vi "prueba.vi"() -> ()   [LabVIEW 2016]
uses:
  <vilib>/userdefined/High Color/IMAQdx.ctl
  <vilib>/UPVI/lvhdf5/file.llb/LVH5F Operation.ctl
  C:/Users/Posgrado/Desktop/Rotational Stage/Thorlabs.MotionControl.Controls.dll
  Rotational Stage/Thorlabs.MotionControl.Controls.dll
  C:/Users/Posgrado/Desktop/Rotational Stage/Thorlabs.MotionControl.IntegratedStepperMotorsCLI.dll
  Rotational Stage/Thorlabs.MotionControl.IntegratedStepperMotorsCLI.dll
  <vilib>/Utility/miscctls.llb/LVRectTypeDef.ctl
  <vilib>/UPVI/lvhdf5/group.llb/H5G_obj_t.ctl
  <vilib>/UPVI/lvhdf5/dataset.llb/LVH5D Operation.ctl
  <vilib>/Analysis/baseanly.llb/Mean (DBL).vi
  <vilib>/UPVI/lvhdf5/group.llb/OpenCreateGroup (String).vi
  <vilib>/UPVI/lvhdf5/utility.llb/Select HDF5 Dialog.vi
  <vilib>/UPVI/lvhdf5/utility.llb/Select HDF5 Dialog (Object Only).vi
  <vilib>/UPVI/lvhdf5/dataset.llb/Simple H5Dwrite (Variant).vi
  <vilib>/UPVI/lvhdf5/library.llb/HDF5 Ref.ctl
  <vilib>/UPVI/lvhdf5/dataset.llb/Simple H5Dwrite.xnode
  <vilib>/vision/driver/NI_Vision_Acquisition_Software.lvlib
  <instrlib>/Keithley 2200 Series/Keithley 2200 Series.lvlib
  <vilib>/Analysis/NI_AALBase.lvlib
  <vilib>/UPVI/lvhdf5/identifier.llb/Not an HDF5 Refnum Constant.vi
  <vilib>/Utility/error.llb/Error Cluster From Error Code.vi
  <vilib>/UPVI/lvhdf5/dataset.llb/OpenCreateReplace Dataset by Element Type.vi
  <vilib>/UPVI/lvhdf5/dataspace.llb/H5Sselect_hyperslab.vi
  <vilib>/UPVI/lvhdf5/dataset.llb/H5Dwrite (Variant).vi
  <vilib>/UPVI/lvhdf5/dataset.llb/H5Dget_space.vi
  <vilib>/UPVI/lvhdf5/attribute.llb/private/LVH5AwriteWDTAttrs.vi
  <vilib>/UPVI/lvhdf5/dataspace.llb/H5Sclose.vi
  <vilib>/UPVI/lvhdf5/dataset.llb/H5Dclose.vi
  <vilib>/UPVI/lvhdf5/utility.llb/Select HDF5 Dialog (File and Object).vi
panel:
  in  "path":path
  out "Ángulo del polarizador":i32
  in  "CageRotatorControl":refnum<k24>(container)
  in  "SerialNumber":string="55000538"
  in  "Ring":u16(ring)
  out "I-V":cluster{dbl[], dbl[]}(graph)
  out "corriente":dbl
  in  "stop medición":bool
  in  "stop":bool
  in  "Iniciar medición":bool
  out "Readout value":dbl format="%^#_9e"
  out "LockIn":dbl
  out "Valor voltaje":dbl
  in  "Config. fotodiodo":cluster{"tiempo. lect.":dbl, "num. med":dbl}
  in  "Powermeter":T1={"Readout Config"="POW", "tiempo. lect."=0.0, "average rate"=0.0}
  in  "config. Polarizador":T2
  in  "Config. voltaje y corriente":T3 {"Measurement Function (0:Voltage)" items=["Voltage", "Current", "Power"]; "Unit(V)" items=["V", "mV", "kV", "A", "mA"]; "Function(0:Voltage)" items=["Voltage", "Current"]}
  in  "yFin":dbl
  in  "Paso":dbl=0.01
  in  "xFin":dbl
  in  "Movimiento de spot en x":ext(slide) scale=-10.0..10.0
  in  "Movimiento de spot en y":dbl(slide) min=-10.0 max=10.0 scale=-10.0..10.0
  out "xsal":dbl
  out "ysal":dbl
  in  "tipo":enum16{"barrido", "manual"}(ring)
  out "Fototubo":cluster{dbl[], dbl[]}(graph)
  out "Power meter":cluster{dbl[], dbl[]}(graph)
  out "Imágen":T4(plugin-control)
  out "flags":bool[](array[boolean])
  out "name":string
  out "Readout string":string
  out "New":bool
  out "Error log":string
  # "Control espejos"
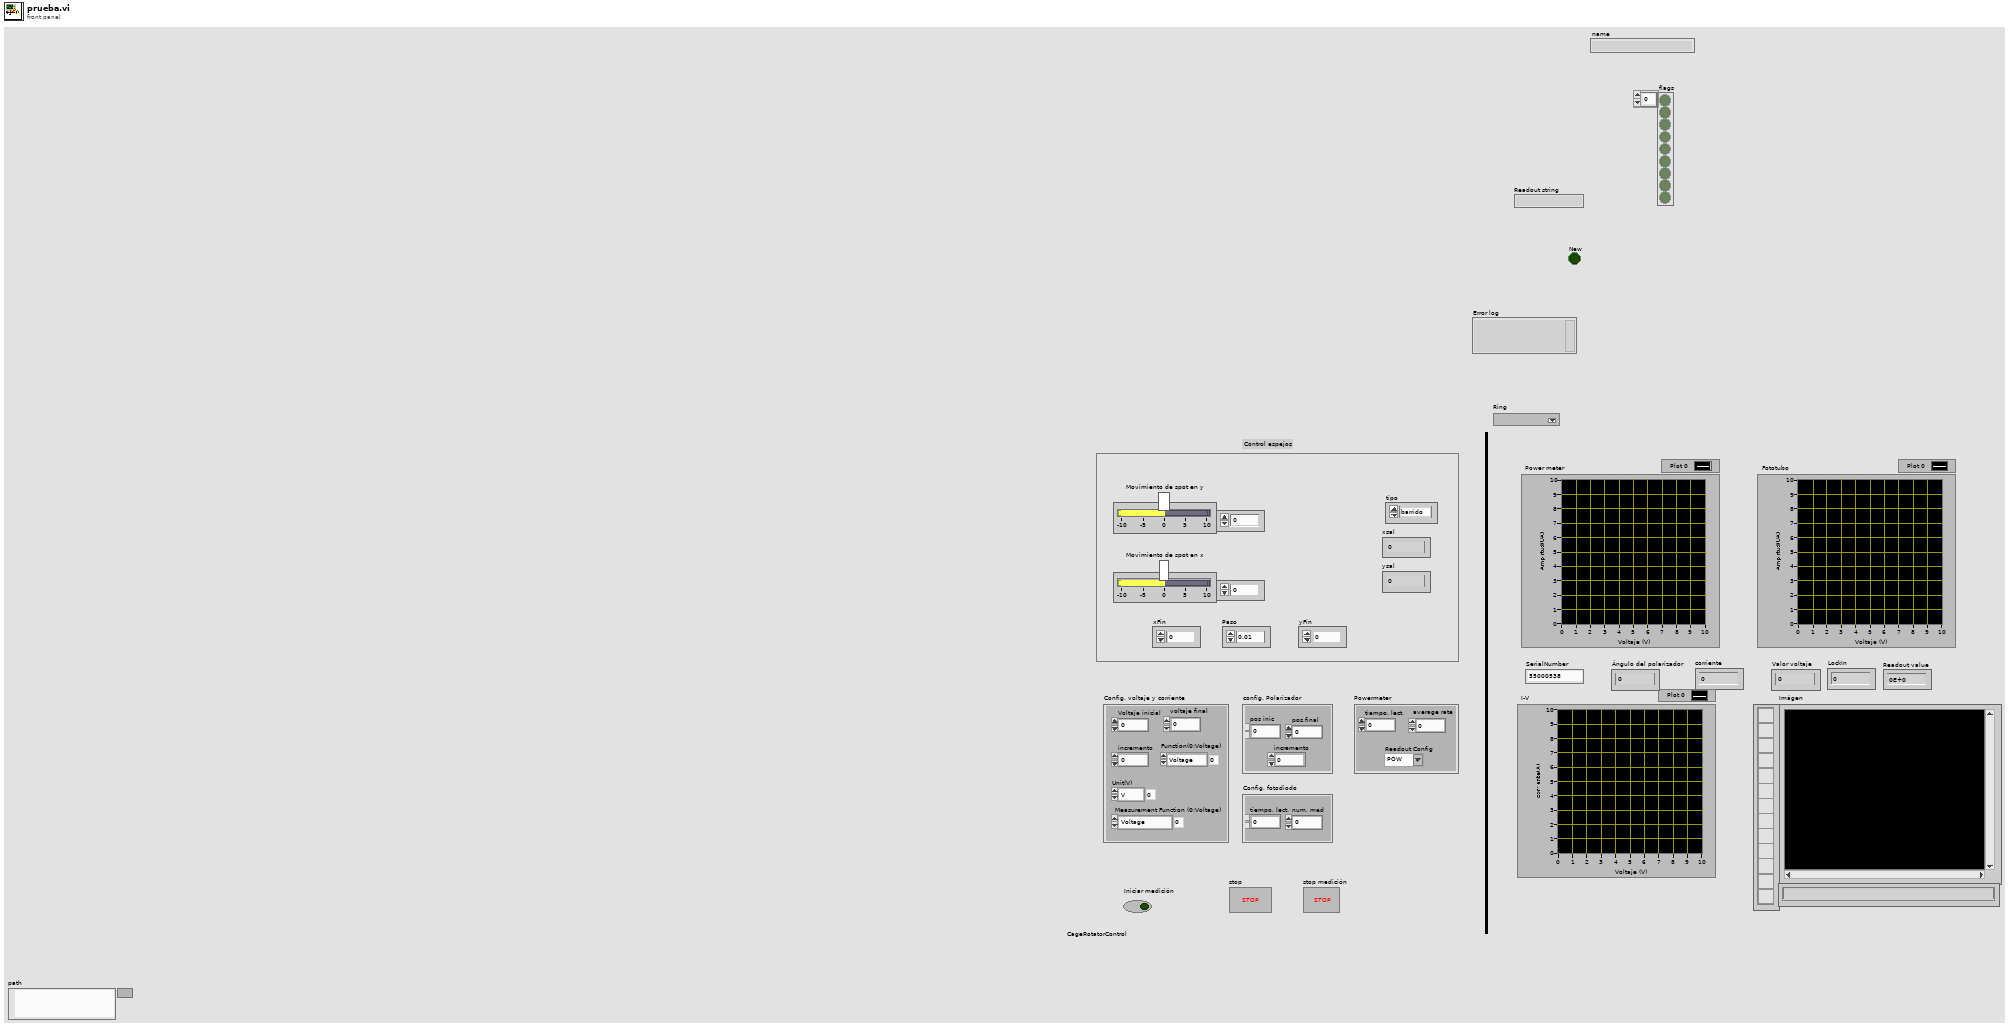
[diagram p1: front panel]
types:
  T1 = cluster{"Readout Config":string, "tiempo. lect.":dbl, "average rate":dbl}
  T2 = cluster{"pos inic":dbl, "pos.final":dbl, "incremento":dbl}
  T3 = cluster{"Voltaje inicial":dbl, "incremento":dbl, " voltaje final":dbl, "Function(0:Voltage)":u16, "Unit(V)":u16, "Measurement Function (0:Voltage)":u16}
  T4 = typedef "IMAQ Image.ctl" = refnum<image>
  T5 = typedef "LVH5F Operation.ctl" = enum16{"open", "open or create", "create or replace", "create or replace (with confirmation)", "create", "open (read only)"}
  T6 = typedef "IMAQdx.ctl" = refnum<k21>
  T7 = typedef "LVRectTypeDef.ctl" = cluster{"Left":i16, "Top":i16, "Right":i16, "Bottom":i16}
  T8 = cluster{"Behavior":enum32{"Invalid", "Default", "Floating", "Floating/Auto-Hide", "Modal"}, "Position":T7, "Center":bool, "Title":string}
  T9 = typedef "LVH5D Operation.ctl" = enum16{"open", "replace", "create", "open or create", "create or replace", "create or replace with confirmation"}
  T10 = typedef "H5G_obj_t.ctl" = i32
  T11 = cluster{"Object Types (any)":T10[], "Object Pattern":string}
  T12 = typedef "Image Type" = u32
  T13 = typedef "HDF5 Ref.ctl" = refnum<k1>
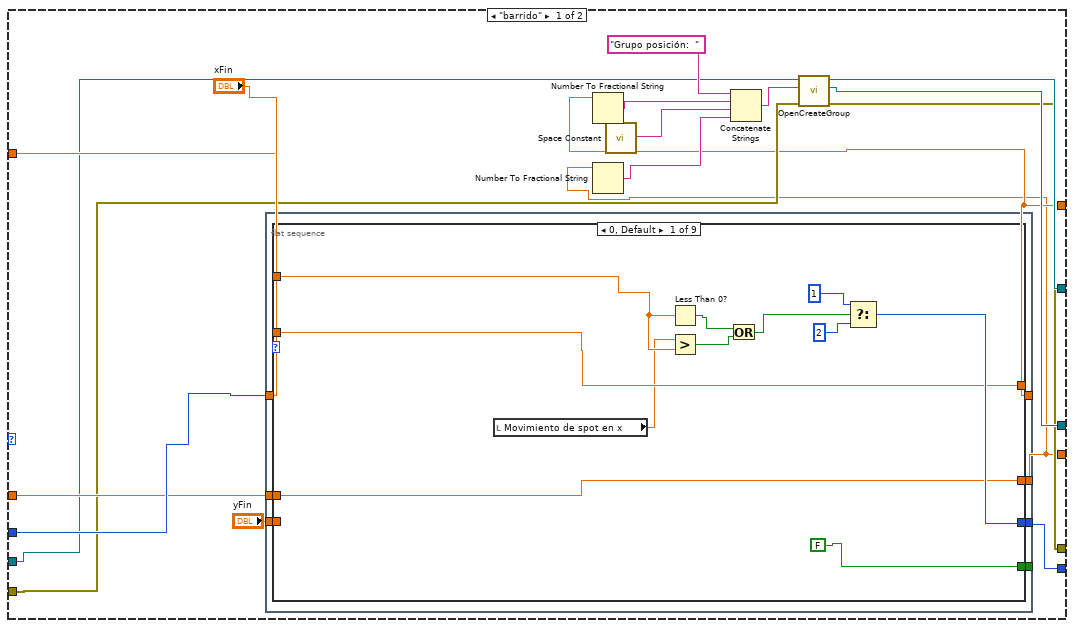
[diagram p2: hidden frame]
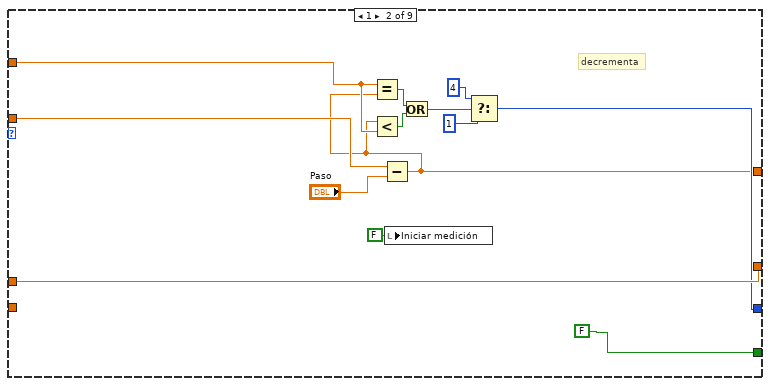
[diagram p3: hidden frame]
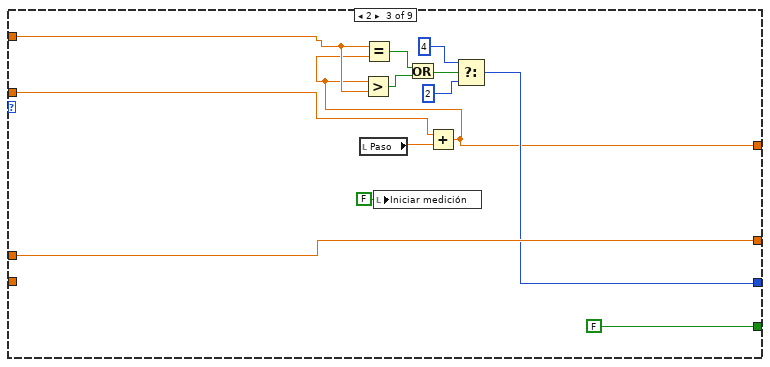
[diagram p4: hidden frame]
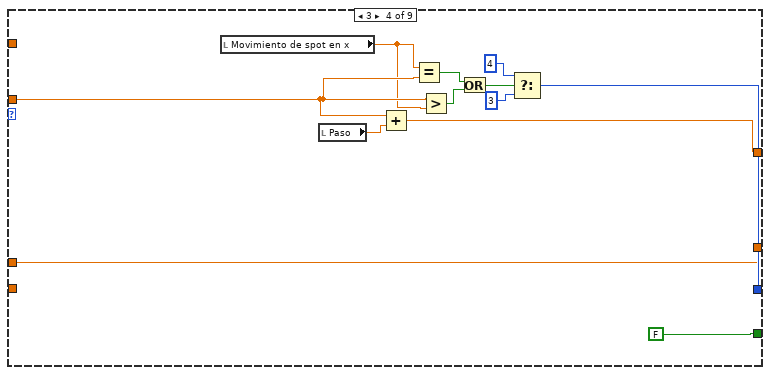
[diagram p5: hidden frame]
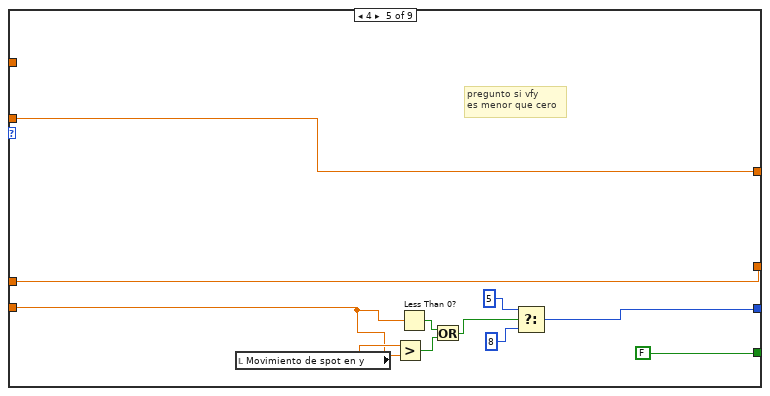
[diagram p6: hidden frame]
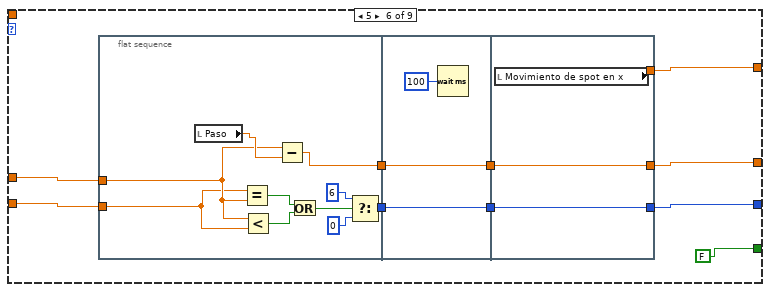
[diagram p7: hidden frame]
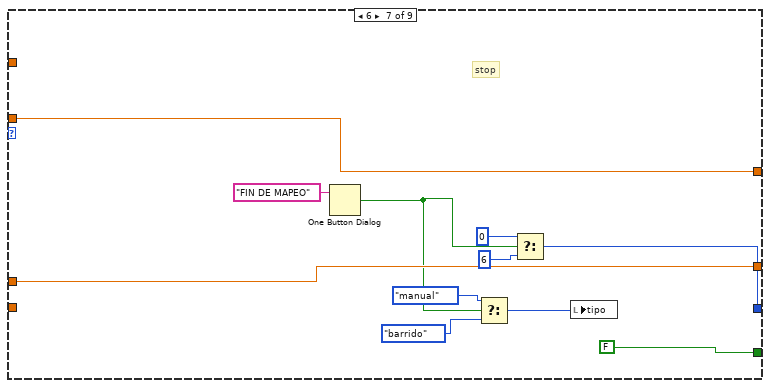
[diagram p8: hidden frame]
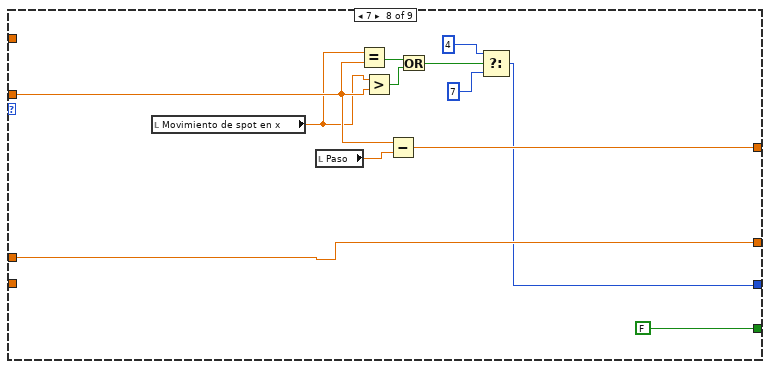
[diagram p9: hidden frame]
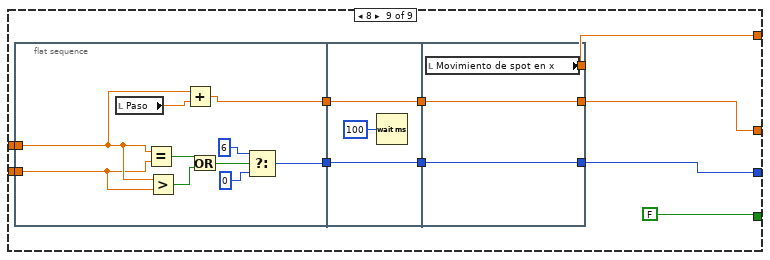
[diagram p10: hidden frame]
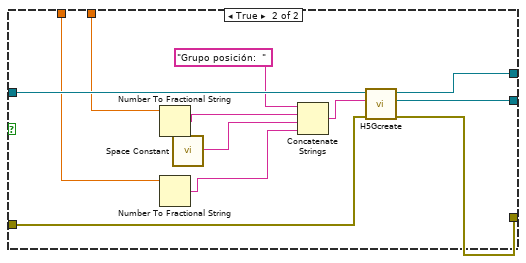
[diagram p11: hidden frame]
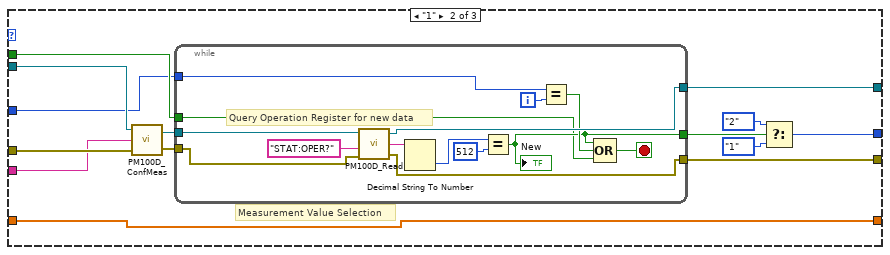
[diagram p13: hidden frame]
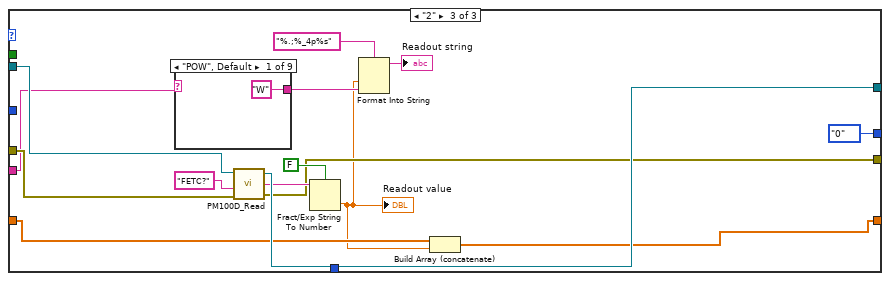
[diagram p14: hidden frame]
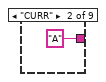
[diagram p15: hidden frame]
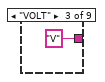
[diagram p16: hidden frame]
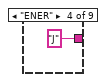
[diagram p17: hidden frame]
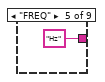
[diagram p18: hidden frame]
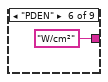
[diagram p19: hidden frame]
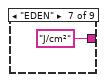
[diagram p20: hidden frame]
diagram:
  n1 = flat-sequence {
    tunnel: [w25] -> w14
    tunnel: [w24] -> w13
    tunnel: [w23] -> w12
    tunnel: [w16] -> w7
    tunnel: [w15] -> w6
    tunnel: w14 -> [w39]
    tunnel: w13 -> [w38]
    tunnel: w12 -> [w37]
    tunnel: [w36] -> w10
    tunnel: [w35] -> w11
    tunnel: [w34] -> w9
    tunnel: w7 -> [w33]
    tunnel: w6 -> [w32]
    tunnel: [w31] -> w5
    tunnel: [w30] -> w4
    tunnel: [w29] -> w3
    frame #0 {
      n2 = call "mapeo.vi"() -> ()  [unwired: 12 in]
    }
    frame #1 {
      w21 = T12 4 items=["Grayscale (U8)", "Grayscale (I16)", "Grayscale (SGL)", "Complex (CSG)", "RGB (U32)", "HSL (U32)", "RGB (U64)", "Grayscale (U16)"] ("Image Type")
      w19 = 5.0
      n3 = call <vilib>:"IMAQdx Open Camera.vi"("Session In"=T6 "cam0") -> ("error out"=w26:errorcluster, "Session Out"=w27:T6)  [unwired: 9 in]
      n4 = call "IMAQ Create"("Image Name"="imagen", "Image Type"=w21) -> ("New Image"=w25:T4)  [unwired: 3 in, 1 out]
      n5 = shared-variable "My Computer\\Library.lvlib\\Vouty"(w19) -> ()  [unwired: 1 in, 1 out]
      n6 = call <vilib>:"OpenCreateReplace HDF5 File.vi"("function (open or create)"=LVH5F_Operation."open or create", "path"="path") -> ("error out"=w15:errorcluster, "HDF5 Ref out"=w16:T13)  [unwired: 6 in]
      n7 = call <vilib>:"IMAQdx Configure Grab.vi"("error in"=w26, "Session In"=w27) -> ("error out"=w23:errorcluster, "Session Out"=w24:T6)  [unwired: 8 in]
      n8 = Wait (ms)(milliseconds to wait=u32 100) -> ()  [unwired: 1 out]
      n9 = shared-variable "My Computer\\Library.lvlib\\Voutx"(w19) -> ()  [unwired: 1 in, 1 out]
      "xsal" <- w19
      "ysal" <- w19
    }
    frame #2 {
      # "error\nfuente de votl"
      # "error\nrot"
      # "error\narchivo"
      n10 = while {
        shift-right: [w70] -> _
        shift-left: _ -> [w67]
        shift-right: [w69] -> _
        shift-left: _ -> [w66]
        shift-right: [w65] -> _
        shift-left: 0 -> [w68]
        tunnel: w39 -> [w58]
        tunnel: w38 -> [w63]
        tunnel: w37 -> [w62]
        tunnel: [w61] -> w36
        tunnel: [w60] -> w35
        tunnel: [w58] -> w34
        tunnel: w33 -> [w53]
        tunnel: w32 -> [w52]
        tunnel: [w43] -> w31
        tunnel: [w42] -> w30
        tunnel: [w41] -> w29
        stop <- "stop" stop-if-true
        # "vy"
        # "vx"
        n11 = call <vilib>:"IMAQdx Grab2.vi"("error in"=w62, "Image In"=w58, "Session In"=w63) -> ("error out"=w60:errorcluster, "Image Out"=→"Imágen":T4, "Session Out"=w61:T6)  [unwired: 5 in, 1 out]
        n12 = flat-sequence {
          tunnel: "tipo" -> [w83]
          tunnel: w68 -> [w82]
          tunnel: w67 -> [w81]
          tunnel: w66 -> [w80]
          tunnel: [w78] -> w56
          tunnel: [w77] -> w55
          tunnel: [w79] -> w54
          tunnel: w53 -> [w76]
          tunnel: w52 -> [w75]
          tunnel: [w74] -> w51
          tunnel: [w73] -> w50
          tunnel: [w72] -> w49
          tunnel: w56 -> [w282]
          tunnel: w55 -> [w281]
          tunnel: w54 -> [w280]
          tunnel: w51 -> [w275]
          tunnel: w50 -> [w274]
          tunnel: w49 -> [w273]
          tunnel: [w282] -> w48
          tunnel: [w281] -> w47
          tunnel: [w280] -> w46
          tunnel: [w272] -> w45
          tunnel: [w271] -> w44
          tunnel: [w270] -> w42
          tunnel: [w269] -> w41
          tunnel: [w932] -> w65
          tunnel: [w933] -> w69
          tunnel: [w934] -> w70
          tunnel: w48 -> [w934]
          tunnel: w47 -> [w933]
          tunnel: w46 -> [w932]
          tunnel: w45 -> [w930]
          tunnel: w44 -> [w931]
          tunnel: [w929] -> w43
          frame #0 {
            # "Movimiento de los espejos"
            # "parte del mapeado"
            n13 = case shown="\"manual\", Default" w83 {
              tunnel: [w85 "Movimiento de spot en x"] -> w78
              tunnel: [w84 "Movimiento de spot en y"] -> w77
              tunnel: w82 -> [w100 w254]
              tunnel: w81 -> [w98 _]
              tunnel: w80 -> [w97 _]
              tunnel: [w96 w254] -> w79
              tunnel: w76 -> [w90 w253]
              tunnel: [w87 w252] -> w73
              tunnel: [w88 w251] -> w74
              tunnel: w75 -> [w89 w248]
              tunnel: [w86 w247] -> w72
              frame "barrido" {
                n14 = flat-sequence {
                  tunnel: "xFin" -> [w110]
                  tunnel: w100 -> [w109]
                  tunnel: [w108] -> w85
                  tunnel: [w107] -> w84
                  tunnel: "yFin" -> [w106]
                  tunnel: w98 -> [w105]
                  tunnel: w97 -> [w104]
                  tunnel: [w103] -> w96
                  tunnel: [w102] -> _
                  frame #0 {
                    n15 = case shown="0, Default" w109 {
                      tunnel: w105 -> [w117 w129 w145 w157 w170 _ w207 w210 _]
                      tunnel: w110 -> [w116 w128 w144 _ _ _ _ _ _]
                      tunnel: w104 -> [w118 w134 w147 w149 w169 w178 w206 w219 w227]
                      tunnel: w106 -> [_ _ _ _ w164 w177 _ _ w226]
                      tunnel: [w120 w130 w140 w151 w167 w180 w202 w216 w228] -> w103
                      tunnel: [w118 w134 w147 w149 w169 w179 w206 w219 w229] -> w107
                      tunnel: [w117 w123 w136 w158 w170 w175 w207 w217 w224] -> w108
                      tunnel: [FALSE FALSE FALSE FALSE ("true") FALSE ("true") FALSE FALSE FALSE ("true") FALSE] -> w102
                      frame 0, Default {
                        n16 = local read "Movimiento de spot en x"() -> (w112:ext)
                        n17 = Less Than 0?(x=w116) -> (x < 0?=w114:bool)
                        n18 = Greater?(x=w112, y=w116) -> (0:w115:bool)
                        n19 = Or(x=w114, y=w115) -> (x .or. y?=w113:bool)
                        n20 = Select(t=1, s=w113, f=2) -> (s? t:f=w120:i32)
                      }
                      frame 1 {
                        # "decrementa"
                        n21 = Subtract(x=w129, y="Paso") -> (x-y=w123:ext)
                        n22 = Equal?(x=w128, y=w123) -> (x = y?=w126:bool)
                        n23 = Less?(x=w123, y=w128) -> (x < y?=w127:bool)
                        n24 = local write "Iniciar medición"(FALSE ("Guarda datos")) -> ()
                        n25 = Or(x=w126, y=w127) -> (x .or. y?=w125:bool)
                        n26 = Select(t=4, s=w125, f=1) -> (s? t:f=w130:i32)
                      }
                      frame 2 {
                        n27 = local read "Paso"() -> (w146:dbl)
                        n28 = local write "Iniciar medición"(FALSE ("Guarda datos")) -> ()
                        n29 = Add(x=w145, y=w146) -> (x+y=w136:ext)
                        n30 = Greater?(x=w136, y=w144) -> (0:w143:bool)
                        n31 = Equal?(x=w144, y=w136) -> (x = y?=w142:bool)
                        n32 = Or(x=w142, y=w143) -> (x .or. y?=w141:bool)
                        n33 = Select(t=4, s=w141, f=2) -> (s? t:f=w140:i32)
                      }
                      frame 3 {
                        n34 = local read "Movimiento de spot en x"() -> (w156:ext)
                        n35 = local read "Paso"() -> (w159:dbl)
                        n36 = Add(x=w157, y=w159) -> (x+y=w158:ext)
                        n37 = Equal?(x=w156, y=w157) -> (x = y?=w154:bool)
                        n38 = Greater?(x=w157, y=w156) -> (0:w155:bool)
                        n39 = Or(x=w154, y=w155) -> (x .or. y?=w153:bool)
                        n40 = Select(t=4, s=w153, f=3) -> (s? t:f=w151:i32)
                      }
                      frame 4 {
                        # "pregunto si vfy\nes menor que cero"
                        n41 = local read "Movimiento de spot en y"() -> (w165:dbl)
                        n42 = Greater?(x=w165, y=w164) -> (0:w162:bool)
                        n43 = Less Than 0?(x=w164) -> (x < 0?=w163:bool)
                        n44 = Or(x=w163, y=w162) -> (x .or. y?=w161:bool)
                        n45 = Select(t=5, s=w161, f=8) -> (s? t:f=w167:i32)
                      }
                      frame 5 {
                        n46 = flat-sequence {
                          tunnel: w178 -> [w183]
                          tunnel: w177 -> [w182]
                          tunnel: [w188] -> w174
                          tunnel: [w186] -> w172
                          tunnel: w174 -> [w193]
                          tunnel: [w193] -> w173
                          tunnel: w172 -> [w192]
                          tunnel: [w192] -> w171
                          tunnel: [w195] -> w179
                          tunnel: [w196] -> w180
                          tunnel: w173 -> [w196]
                          tunnel: w171 -> [w195]
                          tunnel: [w194] -> w175
                          frame #0 {
                            n47 = local read "Paso"() -> (w187:dbl)
                            n48 = Equal?(x=w182, y=w183) -> (x = y?=w184:bool)
                            n49 = Less?(x=w183, y=w182) -> (x < y?=w181:bool)
                            n50 = Subtract(x=w183, y=w187) -> (x-y=w186:dbl)
                            n51 = Or(x=w184, y=w181) -> (x .or. y?=w185:bool)
                            n52 = Select(t=6, s=w185, f=0) -> (s? t:f=w188:i32)
                          }
                          frame #1 {
                            n53 = Wait (ms)(milliseconds to wait=u32 100) -> ()  [unwired: 1 out]
                          }
                          frame #2 {
                            n54 = local read "Movimiento de spot en x"() -> (w194:ext)
                          }
                        }
                      }
                      frame 6 {
                        # "stop"
                        n55 = One Button Dialog(message="FIN DE MAPEO") -> (true=w204:bool)  [unwired: 1 in]
                        n56 = Select(t=enum16{"barrido", "manual"}."manual" ("Enum"), s=w204, f=enum16{"barrido", "manual"}."barrido" ("Enum")) -> (s? t:f=w199:enum16{"barrido", "manual"})
                        n57 = Select(t=0, s=w204, f=6) -> (s? t:f=w202:i32)
                        n58 = local write "tipo"(w199) -> ()
                      }
                      frame 7 {
                        n59 = local read "Movimiento de spot en x"() -> (w208:ext)
                        n60 = local read "Paso"() -> (w218:dbl)
                        n61 = Equal?(x=w208, y=w210) -> (x = y?=w215:bool)
                        n62 = Greater?(x=w208, y=w210) -> (0:w211:bool)
                        n63 = Subtract(x=w210, y=w218) -> (x-y=w217:ext)
                        n64 = Or(x=w215, y=w211) -> (x .or. y?=w214:bool)
                        n65 = Select(t=4, s=w214, f=7) -> (s? t:f=w216:i32)
                      }
                      frame 8 {
                        n66 = flat-sequence {
                          tunnel: w227 -> [w232]
                          tunnel: w226 -> [w231]
                          tunnel: [w238] -> w223
                          tunnel: [w234] -> w221
                          tunnel: w223 -> [w242]
                          tunnel: [w242] -> w222
                          tunnel: w221 -> [w241]
                          tunnel: [w241] -> w220
                          tunnel: [w244] -> w228
                          tunnel: [w245] -> w229
                          tunnel: w222 -> [w245]
                          tunnel: w220 -> [w244]
                          tunnel: [w243] -> w224
                          frame #0 {
                            n67 = local read "Paso"() -> (w239:dbl)
                            n68 = Equal?(x=w232, y=w231) -> (x = y?=w237:bool)
                            n69 = Greater?(x=w232, y=w231) -> (0:w233:bool)
                            n70 = Add(x=w232, y=w239) -> (x+y=w238:dbl)
                            n71 = Or(x=w237, y=w233) -> (x .or. y?=w236:bool)
                            n72 = Select(t=6, s=w236, f=0) -> (s? t:f=w234:i32)
                          }
                          frame #1 {
                            n73 = Wait (ms)(milliseconds to wait=u32 100) -> ()  [unwired: 1 out]
                          }
                          frame #2 {
                            n74 = local read "Movimiento de spot en x"() -> (w243:ext)
                          }
                        }
                      }
                    }
                  }
                }
                n75 = Number To Fractional String(number=w85) -> (F-format string=w93:string)  [unwired: 3 in]
                n76 = Number To Fractional String(number=w84) -> (F-format string=w91:string)  [unwired: 3 in]
                n77 = call <vilib>:"Space Constant.vi"() -> ("String"=w92:string)
                n78 = Concatenate Strings("Grupo posición:  " ("string"), w93, w92, w91) -> (w95:string)
                n79 = call-poly <vilib>:"OpenCreateGroup.vi"("error in (no error)"=w89, "Group"=w95, "HDF5 Ref"=w90) -> ("error out"=w86:errorcluster, "HDF5 Group Ref"=w87:T13, "HDF5 Ref out"=w88:T13)  [unwired: 6 in]
              }
              frame "manual", Default {
                # "referencia"
                # "grupo"
                n80 = local read "Iniciar medición"() -> (w246:bool)
                n81 = case shown="False" w246 {
                  tunnel: w253 -> [w256 w268]
                  tunnel: [_ w267] -> w252
                  tunnel: [w256 w266] -> w251
                  tunnel: "Movimiento de spot en x" -> [_ w263]
                  tunnel: "Movimiento de spot en y" -> [_ w260]
                  tunnel: w248 -> [w255 w258]
                  tunnel: [w255 w257] -> w247
                  frame False {
                  }
                  frame True {
                    n82 = Number To Fractional String(number=w263) -> (F-format string=w262:string)  [unwired: 3 in]
                    n83 = Number To Fractional String(number=w260) -> (F-format string=w259:string)  [unwired: 3 in]
                    n84 = call <vilib>:"Space Constant.vi"() -> ("String"=w261:string)
                    n85 = Concatenate Strings("Grupo posición:  " ("string"), w262, w261, w259) -> (w265:string)
                    n86 = call <vilib>:"H5Gcreate.vi"("error in (no error)"=w258, "Name"=w265, "HDF5 Ref"=w268) -> ("error out"=w257:errorcluster, "HDF5 Group Ref"=w267:T13, "HDF5 Ref out"=w266:T13)  [unwired: 4 in]
                  }
                }
              }
            }
            n87 = local write "ysal"(w77) -> ()
            n88 = local write "xsal"(w78) -> ()
            n89 = shared-variable "My Computer\\Library.lvlib\\Voutx"(w78) -> ()  [unwired: 1 in, 1 out]
            n90 = shared-variable "My Computer\\Library.lvlib\\Vouty"(w77) -> ()  [unwired: 1 in, 1 out]
          }
          frame #1 {
            # "En esta sección se realizan la medición en si"
            n91 = Not Equal?(x=w280, y=4) -> (x != y?=w277:bool)
            n92 = And(x=w277, y="Iniciar medición") -> (x .and. y?=w278:bool)
            n93 = case shown="True" w278 {
              tunnel: w275 -> [w284 w287]
              tunnel: w274 -> [_ w290]
              tunnel: w273 -> [w283 w289]
              tunnel: [w283 w288] -> w272
              tunnel: [w284 w287] -> w271
              tunnel: [_ w286] -> w270
              tunnel: [_ w285] -> w269
              frame False {
              }
              frame True {
                # "archivo"
                n94 = while {
                  shift-right: [w300] -> _
                  shift-left: enum16{"Configurar aparatos", "medir"}."Configurar aparatos" -> [w313]
                  shift-right: [w312] -> w292
                  shift-left: _ -> [w306]
                  shift-right: [w311] -> w291
                  shift-left: _ -> [w305]
                  shift-right: [w310] -> _
                  shift-left: _ -> [w308]
                  shift-right: [w309] -> _
                  shift-left: _ -> [w307]
                  tunnel: refnum<visa-resource-name> refnum ("VISA resource name") -> [w301]
                  tunnel: w290 -> [w299]
                  tunnel: w289 -> [w298]
                  tunnel: [w297] -> w288
                  tunnel: [w296] -> w286
                  tunnel: [w295] -> w285
                  stop <- w304 stop-if-true
                  n95 = case shown="\"medir\"" w313 {
                    tunnel: [w356 w918] -> w312
                    tunnel: [w355 w917] -> w311
                    tunnel: [_ w916] -> w310
                    tunnel: [_ w915] -> w309
                    tunnel: w308 -> [w363 _]
                    tunnel: w307 -> [w362 _]
                    tunnel: w306 -> [w361 _]
                    tunnel: w305 -> [w360 _]
                    tunnel: [TRUE FALSE] -> w302
                    tunnel: w301 -> [w358 _]
                    tunnel: [enum16{"Configurar aparatos", "medir"}."Configurar aparatos" enum16{"Configurar aparatos", "medir"}."medir"] -> w300
                    tunnel: w299 -> [w354 _]
                    tunnel: w298 -> [w353 w910]
                    tunnel: [w316 w910] -> w297
                    tunnel: [w315 _] -> w296
                    tunnel: [w314 _] -> w295
                    frame "medir" {
                      n96 = flat-sequence {
                        tunnel: w353 -> [w374]
                        tunnel: w354 -> [w364]
                        tunnel: w358 -> [w375]
                        tunnel: w360 -> [w376]
                        tunnel: w361 -> [w377]
                        tunnel: w362 -> [w378]
                        tunnel: w363 -> [w379]
                        tunnel: [w379] -> w352
                        tunnel: [w378] -> w351
                        tunnel: [w377] -> w350
                        tunnel: [w376] -> w349
                        tunnel: [w375] -> w348
                        tunnel: [w374] -> w347
                        tunnel: [w367] -> w346
                        tunnel: [w366] -> w345
                        tunnel: [w365] -> w344
                        tunnel: [w364] -> w320
                        tunnel: w352 -> [w392]
                        tunnel: [w392] -> w343
                        tunnel: w351 -> [w391]
                        tunnel: [w391] -> w341
                        tunnel: w350 -> [w390]
                        tunnel: [w390] -> w339
                        tunnel: w349 -> [w389]
                        tunnel: [w389] -> w337
                        tunnel: w348 -> [w388]
                        tunnel: [w388] -> w335
                        tunnel: w347 -> [w387]
                        tunnel: [w387] -> w332
                        tunnel: w346 -> [w386]
                        tunnel: [w386] -> w330
                        tunnel: w345 -> [w384]
                        tunnel: w344 -> [w383]
                        tunnel: [w382] -> w328
                        tunnel: [w381] -> w327
                        tunnel: w320 -> [w380]
                        tunnel: [w380] -> w319
                        tunnel: w343 -> [w409]
                        tunnel: [w409] -> w342
                        tunnel: w341 -> [w408]
                        tunnel: [w408] -> w340
                        tunnel: w339 -> [w407]
                        tunnel: [w407] -> w338
                        tunnel: w337 -> [w406]
                        tunnel: [w406] -> w336
                        tunnel: w335 -> [w405]
                        tunnel: [w405] -> w334
                        tunnel: [w404] -> w333
                        tunnel: w332 -> [w403]
                        tunnel: [w403] -> w331
                        tunnel: w330 -> [w402]
                        tunnel: [w402] -> w329
                        tunnel: w328 -> [w393]
                        tunnel: w327 -> [w401]
                        tunnel: [w395] -> w326
                        tunnel: [w394] -> w325
                        tunnel: w319 -> [w404]
                        tunnel: w342 -> [w426]
                        tunnel: w340 -> [w425]
                        tunnel: w338 -> [w424]
                        tunnel: w336 -> [w423]
                        tunnel: w334 -> [w422]
                        tunnel: w333 -> [w419]
                        tunnel: w331 -> [w418]
                        tunnel: w329 -> [w417]
                        tunnel: w326 -> [w416]
                        tunnel: w325 -> [w415]
                        tunnel: [w421] -> w324
                        tunnel: [w420] -> w323
                        tunnel: [w414] -> w322
                        tunnel: [w413] -> w321
                        tunnel: [w412] -> w318
                        tunnel: [w411] -> w317
                        tunnel: [w410] -> w314
                        tunnel: [w908] -> w355
                        tunnel: [w909] -> w356
                        tunnel: w324 -> [w909]
                        tunnel: w323 -> [w908]
                        tunnel: w322 -> [w907]
                        tunnel: w321 -> [w906]
                        tunnel: w318 -> [w905]
                        tunnel: w317 -> [w904]
                        tunnel: [w903] -> w316
                        tunnel: [w902] -> w315
                        frame #0 {
                          # "inicio de la medición"
                          n97 = property class="CageRotatorControl"(reference="CageRotatorControl", "SerialNumber"="SerialNumber") -> (reference out=w371:refnum<k24>, error out=w370:errorcluster)  [unwired: 1 in]
                          n98 = invoke class="CageRotatorControl" method="CreateDevice"(reference=w371, error in=w370) -> (reference out=w369:refnum<k24>, error out=w368:errorcluster)  [unwired: 1 in, 1 out]
                          n99 = property class="CageRotatorControl"(reference=w369, error in=w368) -> (reference out=w367:refnum<k24>, error out=w365:errorcluster, "Device"=w366:refnum<k24>)
                        }
                        frame #1 {
                          # "timeout"
                          n100 = invoke class="IntegratedStepperMotor" method="Home"(reference=w384, error in=w383, "waitTimeout"=100000 ("Home")) -> (reference out=w382:refnum<k24>, error out=w381:errorcluster)  [unwired: 1 in, 2 out]
                        }
                        frame #2 {
                          # "indica la posición de inicio"
                          n101 = local read "config. Polarizador"() -> (w400:T2)
                          n102 = Unbundle By Name(w400) -> ("pos inic"=w399:dbl)
                          n103 = invoke class="IntegratedStepperMotor" method="SetMoveAbsolutePosition"(reference=w393, error in=w401, "position"=w399) -> (reference out=w398:refnum<k24>, error out=w397:errorcluster)  [unwired: 1 in, 2 out]
                          n104 = invoke class="IntegratedStepperMotor" method="MoveAbsolute"(reference=w398, error in=w397, "waitTimeout"=0) -> (reference out=w395:refnum<k24>, error out=w394:errorcluster)  [unwired: 1 in, 2 out]
                        }
                        frame #3 {
                          # "V"
                          # "grados"
                          n105 = for {
                            tunnel: w426 -> [w445] mode=indexing
                            tunnel: w425 -> [w463]
                            tunnel: w424 -> [w462]
                            tunnel: w423 -> [w461]
                            tunnel: w422 -> [w460]
                            tunnel: [w459] -> w421
                            tunnel: [w458] -> w420
                            tunnel: w419 -> [w456]
                            tunnel: w418 -> [w455]
                            tunnel: w417 -> [w448]
                            tunnel: w416 -> [w447]
                            tunnel: w415 -> [w446]
                            tunnel: [w443] -> w414
                            tunnel: [w442] -> w413
                            tunnel: [w429] -> w412
                            tunnel: [w428] -> w411
                            tunnel: [w427] -> w410
                            stop <- w457 stop-if-true
                            n106 = flat-sequence {
                              tunnel: [w487] -> w454
                              tunnel: [w486] -> w453
                              tunnel: [w485] -> w452
                              tunnel: [w484] -> w451
                              tunnel: [w470] -> w450
                              tunnel: [w483] -> w449
                              tunnel: w463 -> [w487]
                              tunnel: w462 -> [w486]
                              tunnel: w461 -> [w485]
                              tunnel: w460 -> [w484]
                              tunnel: w456 -> [w473]
                              tunnel: w455 -> [w472]
                              tunnel: w448 -> [w483]
                              tunnel: w447 -> [w482]
                              tunnel: w446 -> [w481]
                              tunnel: w445 -> [w467]
                              tunnel: [w474] -> w444
                              tunnel: [w471] -> w441
                              tunnel: [w464] -> w430
                              tunnel: w454 -> [w507]
                              tunnel: w453 -> [w506]
                              tunnel: w452 -> [w505]
                              tunnel: w451 -> [w504]
                              tunnel: w450 -> [w500]
                              tunnel: w449 -> [w498]
                              tunnel: w444 -> [w497]
                              tunnel: w441 -> [w499]
                              tunnel: [w503] -> w440
                              tunnel: [w502] -> w439
                              tunnel: [w498] -> w438
                              tunnel: [w497] -> w437
                              tunnel: [w496] -> w436
                              tunnel: [w495] -> w435
                              tunnel: [w494] -> w434
                              tunnel: [w493] -> w433
                              tunnel: [w492] -> w432
                              tunnel: [w491] -> w431
                              tunnel: w430 -> [w490]
                              tunnel: [w489] -> w429
                              tunnel: [w488] -> w427
                              tunnel: [w696] -> w442
                              tunnel: [w697] -> w443
                              tunnel: [w698] -> w458
                              tunnel: [w699] -> w459
                              tunnel: w440 -> [w699]
                              tunnel: w439 -> [w698]
                              tunnel: w438 -> [w697]
                              tunnel: w437 -> [w696]
                              tunnel: w436 -> [w695]
                              tunnel: w435 -> [w694]
                              tunnel: w434 -> [w693]
                              tunnel: w433 -> [w692]
                              tunnel: w432 -> [w691]
                              tunnel: w431 -> [w690]
                              tunnel: [w686] -> w428
                              frame #0 {
                                # "mover polarizador"
                                n107 = invoke class="IntegratedStepperMotor" method="SetMoveAbsolutePosition"(reference=w482, error in=w481, "position"=w467) -> (reference out=w480:refnum<k24>, error out=w479:errorcluster)  [unwired: 1 in, 2 out]
                                n108 = Number To Fractional String(number=w467) -> (F-format string=w468:string)  [unwired: 3 in]
                                n109 = Concatenate Strings("posición " ("string"), w468, "°" ("string")) -> (w465:string)
                                n110 = invoke class="IntegratedStepperMotor" method="MoveAbsolute"(reference=w480, error in=w479, "waitTimeout"=0) -> (reference out=w477:refnum<k24>, error out=w476:errorcluster)  [unwired: 1 in, 2 out]
                                n111 = call <vilib>:"H5Gcreate.vi"("error in (no error)"=w472, "Name"=w465, "HDF5 Ref"=w473) -> ("error out"=w471:errorcluster, "HDF5 Group Ref"=w470:T13, "HDF5 Ref out"=w464:T13)  [unwired: 4 in]
                                n112 = invoke class="IntegratedStepperMotor" method="GetPositionCounter"(reference=w477, error in=w476) -> (error out=w474:errorcluster, "GetPositionCounter"=→"Ángulo del polarizador":i32)  [unwired: 1 in, 1 out]
                              }
                              frame #1 {
                                w501 = dbl[] []
                                # "Realizar las mediciones de voltale"
                                # "seccion de aduisición de los datos"
                                # "movimiento polarizador"
                                n113 = for {
                                tunnel: w507 -> [w533] mode=indexing
                                tunnel: w506 -> [w531]
                                tunnel: w505 -> [w530]
                                tunnel: w504 -> [w535]
                                shift-right: [w514] -> w494
                                shift-left: w501 -> [w534]
                                shift-right: [w518] -> w493
                                shift-left: w501 -> [w527]
                                shift-right: [w520] -> w492
                                shift-left: w501 -> [w526]
                                tunnel: [w523] -> w503
                                tunnel: [w522] -> w502
                                shift-right: [w515] -> w491
                                shift-left: w501 -> [w517]
                                tunnel: w500 -> [w511]
                                tunnel: w499 -> [w510]
                                tunnel: [w511] -> w496
                                tunnel: [w510] -> w495
                                tunnel: w490 -> [w509]
                                tunnel: [w509] -> w489
                                tunnel: [w508] -> w488
                                stop <- w512 stop-if-true
                                # "potenciometro"
                                # "lockin"
                                # "corriente"
                                # "graficado de datos"
                                # "movimiento voltaje"
                                # "fototubo"
                                # "power"
                                # "voltale"
                                n114 = flat-sequence {
                                tunnel: w533 -> [w546]
                                tunnel: w535 -> [w547]
                                tunnel: [w545] -> w532
                                tunnel: [w539] -> w516
                                tunnel: [w536] -> w508
                                tunnel: w532 -> [w600]
                                tunnel: w531 -> [w596]
                                tunnel: w530 -> [w595]
                                tunnel: [w600] -> _
                                tunnel: [w584] -> w529
                                tunnel: [w583] -> w528
                                tunnel: [w582] -> w523
                                tunnel: [w581] -> w522
                                frame #0 {
                                n115 = local read "Config. voltaje y corriente"() -> (w544:T3)
                                n116 = flat-sequence {
                                tunnel: w547 -> [w566]
                                tunnel: w546 -> [w558]
                                tunnel: w543 -> [w556]
                                tunnel: w542 -> [w555]
                                tunnel: w541 -> [w554]
                                tunnel: [w557] -> w540
                                tunnel: [w549] -> w538
                                tunnel: [w548] -> w537
                                tunnel: [w580] -> w545
                                tunnel: w540 -> [w580]
                                tunnel: [w572] -> w539
                                tunnel: w538 -> [w571]
                                tunnel: w537 -> [w579]
                                tunnel: [w570] -> w536
                                frame #0 {
                                # "obtener valor  del voltaje"
                                n117 = call <instrlib>:"Initialize.vi"("VISA resource name"=w566) -> ("error out"=w564:errorcluster, "VISA resource name out"=w565:refnum<visa-resource-name>)  [unwired: 9 in]
                                n118 = call <instrlib>:"Configure Output.vi"("VISA resource name"=w565, "Manual Range(0.00)"=w558, "Function(0:Voltage)"=w556, "Enable Output (T: Enable)"=TRUE, "error in (no error)"=w564, "Unit(V)"=w555) -> ("VISA resource name out"=w562:refnum<visa-resource-name>, "error out"=w561:errorcluster)  [unwired: 8 in]
                                n119 = flat-sequence {
                                tunnel: w561 -> [w568]
                                tunnel: [w568] -> w560
                                tunnel: w562 -> [w567]
                                tunnel: [w567] -> w549
                                frame #0 {
                                n120 = Wait (ms)(milliseconds to wait=u32 1000) -> ()  [unwired: 1 out]
                                }
                                }
                                n121 = call <instrlib>:"Read Output.vi"("VISA resource name"=w549, "Measurement Function (0:Voltage)"=w554, "error in (no error)"=w560) -> ("VISA resource name out"=w553:refnum<visa-resource-name>, "Measurement"=w559:string, "error out"=w552:errorcluster)  [unwired: 10 in]
                                n122 = Fract/Exp String To Number(string=w559) -> (number=w557:dbl)  [unwired: 3 in, 1 out]
                                "Valor voltaje" <- w557
                                n123 = call <instrlib>:"Error Query.vi"("error in (no error)"=w552, "VISA resource name"=w553) -> ("error out"=w551:errorcluster, "VISA resource name out"=w550:refnum<visa-resource-name>)  [unwired: 6 in, 2 out]
                                n124 = call <instrlib>:"Close.vi"("error in (no error)"=w551, "VISA resource name"=w550) -> ("error out"=w548:errorcluster)  [unwired: 9 in]
                                }
                                frame #1 {
                                w578 = u16 1 items=["Voltage", "Current", "Power"] ("Measurement Function (0:Voltage)")
                                n125 = call <instrlib>:"Read Output.vi"("VISA resource name"=w571, "Measurement Function (0:Voltage)"=w578, "error in (no error)"=w579) -> ("VISA resource name out"=w574:refnum<visa-resource-name>, "Measurement"=w577:string, "error out"=w573:errorcluster)  [unwired: 10 in]
                                n126 = Fract/Exp String To Number(string=w577) -> (number=w572:dbl)  [unwired: 3 in, 1 out]
                                "corriente" <- w572
                                n127 = call <instrlib>:"Error Query.vi"("error in (no error)"=w573, "VISA resource name"=w574) -> ("error out"=w575:errorcluster, "VISA resource name out"=w576:refnum<visa-resource-name>)  [unwired: 6 in, 2 out]
                                n128 = call <instrlib>:"Close.vi"("error in (no error)"=w575, "VISA resource name"=w576) -> ("error out"=w570:errorcluster)  [unwired: 9 in]
                                }
                                }
                                n129 = Unbundle By Name(w544) -> ("Function(0:Voltage)"=w543:u16, "Unit(V)"=w542:u16, "Measurement Function (0:Voltage)"=w541:u16)
                                }
                                frame #1 {
                                # "adquisición"
                                n130 = local read "Config. fotodiodo"() -> (w599:cluster{"tiempo. lect.":dbl, "num. med":dbl})
                                n131 = local read "Powermeter"() -> (w592:T1)
                                n132 = Unbundle By Name(w592) -> ("Readout Config"=w591:string, "tiempo. lect."=w590:dbl, "average rate"=w588:dbl)
                                n133 = To Long Integer(number=w588) -> (32bit integer=w587:i32)
                                n134 = To Long Integer(number=w590) -> (32bit integer=w589:i32)
                                n135 = Unbundle By Name(w599) -> ("tiempo. lect."=w598:dbl, "num. med"=w597:dbl)
                                n136 = To Long Integer(number=w597) -> (32bit integer=w586:i32)
                                n137 = To Long Integer(number=w598) -> (32bit integer=w585:i32)
                                n138 = for {
                                N: w586 -> [w616]
                                shift-right: [w603] -> _
                                shift-left: enum16{"0", "1", "2"}."0" -> [w618]
                                tunnel: w596 -> [w620]
                                tunnel: w595 -> [w619]
                                shift-right: [w613] -> w584
                                shift-left: dbl[] [] -> [w612]
                                tunnel: [w610] -> w583 mode=indexing
                                tunnel: w591 -> [w609]
                                tunnel: w589 -> [w608]
                                tunnel: w587 -> [w607]
                                tunnel: w585 -> [w606]
                                tunnel: [w605] -> w582
                                tunnel: [w604] -> w581
                                i -> [w615]
                                w611 = u16 0 items=["LockIn", "LockIn-DMM"] ("Tipo")
                                n139 = Increment(x=w615) -> (x+1=w614:i32)
                                n140 = Wait (ms)(milliseconds to wait=w606) -> ()  [unwired: 1 out]
                                n141 = Greater Or Equal?(x=w616, y=w614) -> (x >= y?=w617:bool)
                                n142 = call "25_P-GPIB-LockIn510.vi"("Tipo"=w611, "P-DMM"="1:16", "P-LockIn"="1:3") -> ("LockIn"=w610:dbl)  [unwired: 1 in, 1 out]
                                "LockIn" <- w610
                                n143 = case shown="\"0\", Default" w618 {
                                tunnel: w620 -> [w631 w647 w674]
                                tunnel: w619 -> [w626 w646 w673]
                                tunnel: [enum16{"0", "1", "2"}."1" w641 enum16{"0", "1", "2"}."0"] -> w603
                                tunnel: [w624 w643 w672] -> w605
                                tunnel: [w623 w642 w666] -> w604
                                tunnel: w617 -> [_ w637 _]
                                tunnel: w612 -> [w622 w636 w665]
                                tunnel: [w622 w636 w663] -> w613
                                tunnel: w609 -> [_ w635 w662]
                                tunnel: w608 -> [_ w634 _]
                                tunnel: w607 -> [w621 _ _]
                                frame "0", Default {
                                # "Query errors"
                                # "Example: setting the averaging rate"
                                # "Measurement Configuration\nUse this frame to set the measurement relevant parameters\ne.g. wavelength, measurement range, bandwidth etc."
                                n144 = Number To Decimal String(number=w621) -> (decimal integer string=w632:string)  [unwired: 1 in]
                                n145 = Concatenate Strings("SENS:AVER " ("string"), w632) -> (w630:string)
                                n146 = call "PM100D_Write.vi"("error in (no error)"=w626, "Command"=w630, "VISA in"=w631) -> ("error out"=w627:errorcluster, "VISA out"=w629:refnum<visa-resource-name>)
                                n147 = call "PM100D_SYST-ERR.vi"("error out 2"=w627, "VISA In"=w629) -> ("error out"=w623:errorcluster, "Error"=→"Error log":string, "VISA Out"=w624:refnum<visa-resource-name>)  [unwired: 1 in]
                                }
                                frame "1" {
                                # "Measurement Value Selection"
                                n148 = call "PM100D_ConfMeas.vi"("error in"=w646, "Conf:"=w635, "VISA In"=w647) -> ("error out"=w644:errorcluster, "dup VISA session"=w645:refnum<visa-resource-name>)
                                n149 = while {
                                tunnel: w645 -> [w657]
                                tunnel: w644 -> [w656]
                                tunnel: [w655] -> w643
                                tunnel: [w654] -> w642
                                tunnel: [w650] -> w638
                                tunnel: w637 -> [w649]
                                tunnel: w634 -> [w648]
                                i -> [w652]
                                stop <- w653 stop-if-true
                                # "Query Operation Register for new data"
                                n150 = call "PM100D_Read.vi"("error in (no error)"=w656, "Command"="STAT:OPER?", "VISA in"=w657) -> ("error out"=w654:errorcluster, "ReadValue"=w660:string, "VISA out"=w655:refnum<visa-resource-name>)  [unwired: 1 in]
                                n151 = Decimal String To Number(string=w660) -> (number=w659:i32)  [unwired: 2 in, 1 out]
                                n152 = Equal?(x=w659, y=512) -> (x = y?=w650:bool)
                                "New" <- w650
                                n153 = Equal?(x=w648, y=w652) -> (x = y?=w651:bool)
                                n154 = Compound Arithmetic op=OR(w650, w651, w649) -> (w653:bool)
                                }
                                n155 = Select(t=enum16{"0", "1", "2"}."2", s=w638, f=enum16{"0", "1", "2"}."1") -> (s? t:f=w641:enum16{"0", "1", "2"})
                                }
                                frame "2" {
                                n156 = case shown="\"POW\", Default" w662 {
                                tunnel: ["W" "A" "V" "J" "Hz" "W/cm²" "J/cm²" "Ohm" "°C"] -> w668
                                frame "POW", Default {
                                }
                                frame "CURR" {
                                }
                                frame "VOLT" {
                                }
                                frame "ENER" {
                                }
                                frame "FREQ" {
                                }
                                frame "PDEN" {
                                }
                                frame "EDEN" {
                                }
                                frame "RES" {
                                }
                                frame "TEMP" {
                                }
                                }
                                n157 = call "PM100D_Read.vi"("error in (no error)"=w673, "Command"="FETC?", "VISA in"=w674) -> ("error out"=w666:errorcluster, "ReadValue"=w671:string, "VISA out"=w672:refnum<visa-resource-name>)  [unwired: 1 in]
                                n158 = Fract/Exp String To Number(use system decimal point (T)=FALSE, string=w671) -> (number=w664:dbl)  [unwired: 2 in, 1 out]
                                "Readout value" <- w664
                                n159 = Format Into String(format string="%.;%_4p%s", w664, w668) -> (resulting string=→"Readout string":string)  [unwired: 2 in, 1 out]
                                n160 = Build Array (concatenate)(w665, w664) -> (w663:dbl[])
                                }
                                }
                                }
                                }
                                }
                                n161 = Build Array (concatenate)(w534, w533) -> (w514:dbl[])
                                n162 = Build Array (concatenate)(w517, w516) -> (w515:dbl[])
                                n163 = call-poly <vilib>:"Mean.vi"("X"=w529) -> ("mean"=w525:dbl)  [unwired: 1 out]
                                n164 = call-poly <vilib>:"Mean.vi"("X"=w528) -> ("mean"=w524:dbl)  [unwired: 1 out]
                                n165 = Build Array (concatenate)(w527, w525) -> (w518:dbl[])
                                n166 = Build Array (concatenate)(w526, w524) -> (w520:dbl[])
                                n167 = local read "stop medición"() -> (w512:bool)
                                n168 = Bundle(w514, w515) -> (→"I-V":cluster{dbl[], dbl[]})  [unwired: 1 in]
                                n169 = Bundle(w514, w518) -> (→"Fototubo":cluster{dbl[], dbl[]})  [unwired: 1 in]
                                n170 = Bundle(w514, w520) -> (→"Power meter":cluster{dbl[], dbl[]})  [unwired: 1 in]
                                }
                              }
                              frame #2 {
                                # "Guardado de datos"
                                n171 = Build Array(w693, w692, w691, w690) -> (w689:dbl[][])
                                n172 = xnode "Simple H5Dwrite"("error in (no error)"=w694, "HDF5 Path or Ref"=w695, "Data"=w689) -> ("HDF5 Ref out"=w688:T13, "error out"=w687:errorcluster)  [unwired: 5 in, 1 out]
                                n173 = call <vilib>:"H5Gclose.vi"("error in (no error)"=w687, "HDF5 Group Ref"=w688) -> ("error out"=w686:errorcluster)  [unwired: 7 in]
                              }
                            }
                            n174 = local read "stop medición"() -> (w457:bool)
                          }
                        }
                        frame #4 {
                          n175 = invoke class="CageRotatorControl" method="CloseDevice"(reference=w907, error in=w906) -> (error out=w902:errorcluster)  [unwired: 1 in, 2 out]
                          n176 = call <vilib>:"H5Gclose.vi"("error in (no error)"=w904, "HDF5 Group Ref"=w905) -> ("error out"=w903:errorcluster)  [unwired: 7 in]
                        }
                      }
                    }
                    frame "Configurar aparatos" {
                      # "fuente de voltaje"
                      # "Powermeter"
                      n177 = local read "Config. voltaje y corriente"() -> (w913:T3)
                      n178 = local read "config. Polarizador"() -> (w914:T2)
                      n179 = Unbundle By Name(w913) -> ("Voltaje inicial"=w921:dbl, "incremento"=w920:dbl, "voltaje final"=w919:dbl)
                      n180 = Unbundle By Name(w914) -> ("pos inic"=w923:dbl, "pos.final"=w922:dbl, "incremento"=w924:dbl)
                      n181 = call "PM100D_Initialize.vi"() -> ("error out"=w927:errorcluster, "VISA out"=w928:refnum<visa-resource-name>)  [unwired: 2 in, 2 out]
                      n182 = call "PM100D_SensorFlag.vi"("error in (no error)"=w927, "VISA in"=w928) -> ("error out"=w917:errorcluster, "flags"=→"flags":bool[], "VISA out"=w918:refnum<visa-resource-name>, "name"=→"name":string)  [unwired: 2 in, 4 out]
                      n183 = call "intervalo.vi"("incremento"=w924, "fin"=w922, "inicio"=w923) -> ("Array"=w916:dbl[])  [unwired: 8 in]
                      n184 = call "intervalo.vi"("incremento"=w919, "fin"=w920, "inicio"=w921) -> ("Array"=w915:dbl[])  [unwired: 8 in]
                    }
                  }
                  n185 = Or(x=w302, y="stop medición") -> (x .or. y?=w304:bool)
                }
                n186 = call "PM100D_Close.vi"("error in (no error)"=w291, "VISA resource name"=w292) -> ()  [unwired: 2 in]
              }
            }
          }
          frame #2 {
            # "cierra archivo"
            n187 = call <vilib>:"H5Fclose.vi"("error in (no error)"=w930, "HDF5 Ref"=w931) -> ("error out"=w929:errorcluster)  [unwired: 7 in]
          }
        }
        n188 = Wait (ms)(milliseconds to wait=u32 400) -> ()  [unwired: 1 out]
        n189 = shared-variable "NI-cRIO9074\\Library_CRIO.lvlib\\Stop_read"("stop") -> ()  [unwired: 1 in, 1 out]
      }
    }
  }
  n190 = call <vilib>:"IMAQdx Close Camera.vi"("error in"=w11, "Session In"=w10) -> ("error out"=w8:errorcluster)  [unwired: 9 in]
  n191 = call "IMAQ Dispose"("Image"=w9, "error in (no error)"=w8) -> ("error out"=w2:errorcluster)  [unwired: 4 in]
  n192 = Merge Errors(w4, w3, w5, w2) -> (w1:errorcluster)
  n193 = call <vilib>:"General Error Handler.vi"("error in (no error)"=w1) -> ()  [unwired: 10 in, 5 out]
